vi "set UI state when start line.vi"(7 "start?":bool=TRUE, 9 "index of element":i32, 10 "UI Refs":T4) -> (1 "start info - logging loop":T3, 2 "start info - digital control loop":T1)   [LabVIEW 2014]
uses:
  controls/PLS UI Data.ctl
  Digital Control/type de test.ctl
  Logging/start info.ctl
  Digital Control/start info.ctl
  Logging/PLS Logging.lvlib
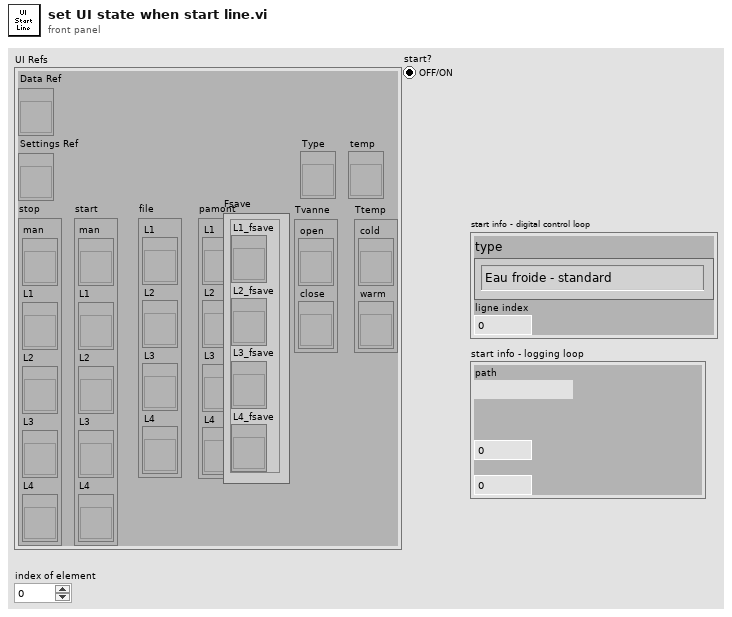
[diagram p1: front panel]
types:
  T1 = typedef "start info.ctl" = cluster{"type":T2, "ligne index":i32}
  T2 = typedef "type de test.ctl" = enum16{"Eau froide - standard", "Eau chaude", "Chocs thermiques"}
  T3 = typedef "PLS Logging.lvlib/start info.ctl" = cluster{"path":path, "Fsave":i32, "#ligne":i32}
  T4 = typedef "PLS UI Data.ctl" = cluster{"Data Ref":refnum<vi>, "Settings Ref":refnum<vi>, "stop":cluster{"man":refnum<vi>, "L1":refnum<vi>, "L2":refnum<vi>, "L3":refnum<vi>, "L4":refnum<vi>}, "start":cluster{"man":refnum<vi>, "L1":refnum<vi>, "L2":refnum<vi>, "L3":refnum<vi>, "L4":refnum<vi>}, "file":cluster{"L1":refnum<vi>, "L2":refnum<vi>, "L3":refnum<vi>, "L4":refnum<vi>}, "pamont":cluster{"L1":refnum<vi>, "L2":refnum<vi>, "L3":refnum<vi>, "L4":refnum<vi>}, "Fsave":cluster{"L1_fsave":refnum<vi>, "L2_fsave":refnum<vi>, "L3_fsave":refnum<vi>, "L4_fsave":refnum<vi>}, "Tvanne":cluster{"open":refnum<vi>, "close":refnum<vi>}, "Ttemp":cluster{"cold":refnum<vi>, "warm":refnum<vi>}, "temp":refnum<vi>, "Type":refnum<vi>}
  T5 = cluster{"L1_fsave":refnum<vi>, "L2_fsave":refnum<vi>, "L3_fsave":refnum<vi>, "L4_fsave":refnum<vi>}
  T6 = cluster{"L1":refnum<vi>, "L2":refnum<vi>, "L3":refnum<vi>, "L4":refnum<vi>}
  T7 = cluster{"man":refnum<vi>, "L1":refnum<vi>, "L2":refnum<vi>, "L3":refnum<vi>, "L4":refnum<vi>}
  T8 = enum16{"Eau froide - standard", "Eau chaude", "Chocs thermiques"}
  T9 = enum16{"open", "replace", "create", "open or create", "replace or create", "replace or create with confirmation"}
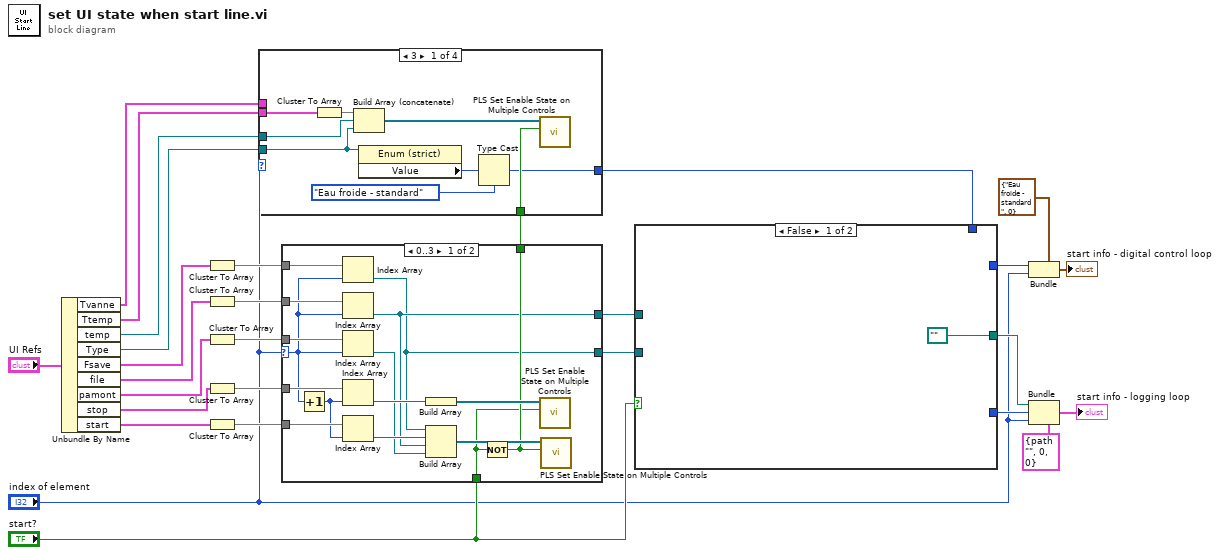
[diagram p0: block diagram]
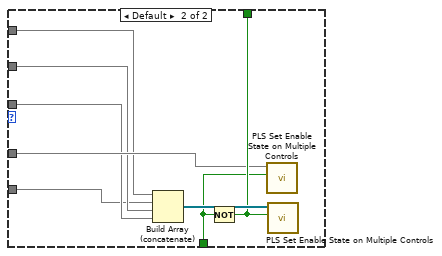
[diagram p2: hidden frame]
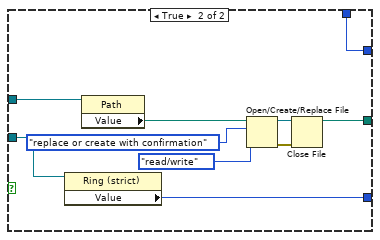
[diagram p3: hidden frame]
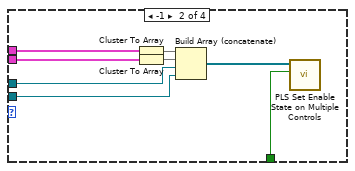
[diagram p4: hidden frame]
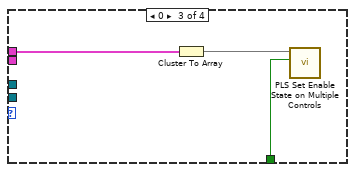
[diagram p5: hidden frame]
diagram:
  n1 = Unbundle By Name("UI Refs") -> ("Tvanne"=w15:cluster{"open":refnum<vi>, "close":refnum<vi>}, "Ttemp"=w16:cluster{"cold":refnum<vi>, "warm":refnum<vi>}, "temp"=w17:refnum<vi>, "Type"=w13:refnum<vi>, "Fsave"=w18:T5, "file"=w21:T6, "pamont"=w20:T6, "stop"=w25:T7, "start"=w26:T7)
  n2 = Cluster To Array(cluster=w18) -> (array=w19:refnum<vi>[])
  n3 = Cluster To Array(cluster=w21) -> (array=w22:refnum<vi>[])
  n4 = Cluster To Array(cluster=w20) -> (array=w23:refnum<vi>[])
  n5 = Cluster To Array(cluster=w25) -> (array=w28:refnum<vi>[])
  n6 = Cluster To Array(cluster=w26) -> (array=w27:refnum<vi>[])
  n7 = case shown="0..3" "index of element" {
    selector: "index of element" -> [w29 _]
    tunnel: w28 -> [w40 w49]
    tunnel: w27 -> [w39 w45]
    tunnel: w23 -> [w38 w46]
    tunnel: w22 -> [w37 w47]
    tunnel: w19 -> [w36 w48]
    tunnel: [w35 w51] -> w14
    tunnel: [w34 _] -> w12
    tunnel: "start?" -> [w33 w50]
    tunnel: [w31 _] -> w10
    frame 0..3 {
      n8 = Increment(x=w29) -> (x+1=w30:i32)
      n9 = Index Array(array=w36, index=w29) -> (element=w31:refnum<vi>)
      n10 = Index Array(array=w37, index=w29) -> (element=w34:refnum<vi>)
      n11 = Index Array(array=w38, index=w29) -> (element=w32:refnum<vi>)
      n12 = Index Array(array=w40, index=w30) -> (element=w41:refnum<vi>)
      n13 = Index Array(array=w39, index=w30) -> (element=w43:refnum<vi>)
      n14 = Build Array(w41) -> (w42:refnum<vi>[])
      n15 = Build Array(w31, w43, w34, w32) -> (w44:refnum<vi>[])
      n16 = Not(x=w33) -> (.not. x?=w35:bool)
      n17 = call "PLS Set Enable State on Multiple Controls.vi"("Enable?"=w33, "Controls"=w42) -> ()  [unwired: 10 in]
      n18 = call "PLS Set Enable State on Multiple Controls.vi"("Enable?"=w35, "Controls"=w44) -> ()  [unwired: 10 in]
    }
    frame Default {
      n19 = Build Array (concatenate)(w48, w45, w47, w46) -> (w52:refnum<vi>[])
      n20 = Not(x=w50) -> (.not. x?=w51:bool)
      n21 = call "PLS Set Enable State on Multiple Controls.vi"("Enable?"=w50, "Controls"=w49) -> ()  [unwired: 10 in]
      n22 = call "PLS Set Enable State on Multiple Controls.vi"("Enable?"=w51, "Controls"=w52) -> ()  [unwired: 10 in]
    }
  }
  n23 = case shown="3" "index of element" {
    tunnel: w17 -> [w58 w66 _ _]
    tunnel: w16 -> [w61 w69 _ _]
    tunnel: w15 -> [_ w63 w71 _]
    tunnel: w14 -> [w57 w65 w70 _]
    tunnel: w13 -> [w56 w64 _ _]
    tunnel: [w53 _ _ _] -> w5
    frame 3 {
      n24 = Cluster To Array(cluster=w61) -> (array=w60:refnum<vi>[])
      n25 = Build Array (concatenate)(w60, w58, w56) -> (w59:refnum<vi>[])
      n26 = property class="Enum (strict)"(reference=w56) -> ("Value"=w55:T8)  [unwired: 1 in, 2 out]
      n27 = Type Cast(type=type_de_test."Eau froide - standard" ("Value"), x=w55) -> (*(type *) &x=w53:T2)
      n28 = call "PLS Set Enable State on Multiple Controls.vi"("Enable?"=w57, "Controls"=w59) -> ()  [unwired: 10 in]
    }
    frame -1 {
      n29 = Cluster To Array(cluster=w63) -> (array=w62:refnum<vi>[])
      n30 = Cluster To Array(cluster=w69) -> (array=w68:refnum<vi>[])
      n31 = Build Array (concatenate)(w62, w68, w66, w64) -> (w67:refnum<vi>[])
      n32 = call "PLS Set Enable State on Multiple Controls.vi"("Enable?"=w65, "Controls"=w67) -> ()  [unwired: 10 in]
    }
    frame 0 {
      n33 = Cluster To Array(cluster=w71) -> (array=w72:refnum<vi>[])
      n34 = call "PLS Set Enable State on Multiple Controls.vi"("Enable?"=w70, "Controls"=w72) -> ()  [unwired: 10 in]
    }
    frame Default {
    }
  }
  n35 = case shown="False" "start?" {
    tunnel: w12 -> [_ w83]
    tunnel: [path "" ("path") w77] -> w9
    tunnel: w10 -> [_ w76]
    tunnel: [_ w75] -> w8
    tunnel: w5 -> [_ w74]
    tunnel: [_ w74] -> w4
    frame False {
    }
    frame True {
      n36 = property class="Ring (strict)"(reference=w76) -> ("Value"=w75:i32)  [unwired: 1 in, 2 out]
      n37 = property class="Path"(reference=w83) -> ("Value"=w82:path)  [unwired: 1 in, 2 out]
      n38 = Open/Create/Replace File(file path (use dialog)=w82, operation (0:open)=T9."replace or create with confirmation", access (0:read/write)=enum16{"read/write", "read-only", "write-only"}."read/write") -> (refnum out=w79:refnum<file>, error out=w80:errorcluster)  [unwired: 3 in, 1 out]
      n39 = Close File(refnum=w79, error in=w80) -> (path=w77:path)  [unwired: 1 out]
    }
  }
  n40 = Bundle(cluster=T1 {"type"=enum."Eau froide - standard", "ligne index"=0} ("start info"), "type"=w4, "ligne index"="index of element") -> (→"start info - digital control loop":T1)
  n41 = Bundle(cluster=T3 {"path"=path "", "Fsave"=0, "#ligne"=0} ("start info"), "path"=w9, "Fsave"=w8, "#ligne"="index of element") -> (→"start info - logging loop":T3)
